vi "Control BrakeCoast[Conflict].vi"   [LabVIEW 2017]
uses:
  <vilib>/Rock Robotics/WPI/ThirdParty/Phoenix-LabVIEW/Motor Controller/Controls/CTRE_Phoenix_MotorControl_NeutralMode.ctl
types:
  T1 = cluster{"LinearAcceleration X":dbl, "LinearAcceleration Y":dbl, "LinearAcceleration Z":dbl}
  T2 = typedef "WPI_MotorControlDeviceRef.ctl" = cluster{"DeviceStatus":errorcluster, "Type":T3, "PWM":cluster{"PWM Channel":T4, "DeadBand":T5}, "CAN":cluster{"Device Number":u8, "SetOutput VI Ref":variant, "GetOutput VI Ref":variant, "Enable VI Ref":variant, "Disable VI Ref":variant, "Data":variant}, "Invert":bool, "DIO PWM":cluster{"PWM \"Enable\" Channel":T4, "DIOChannel":T6, "PWM Rate":dbl}}
  T3 = typedef "WPI_MotorControlType.ctl" = enum16{"PWM", "CAN", "DIO PWM"}
  T4 = typedef "FPGA_DIOPWMChannel.ctl" = enum8{"PWM 0", "PWM 1", "PWM 2", "PWM 3", "PWM 4", "PWM 5", "PWM 6", "PWM 7", "PWM 8", "PWM 9", "PWM MXP 0", "PWM MXP 1", "PWM MXP 2", "PWM MXP 3", "PWM MXP 4", "PWM MXP 5", "PWM MXP 6", "PWM MXP 7", "PWM MXP 8", "PWM MXP 9", "Invalid"}
  T5 = typedef "WPI_PWMDeadband.ctl" = cluster{"Name":string, "maxPositivePwm":i32, "minPositivePwm":i32, "centerPwm":i32, "maxNegativePwm":i32, "minNegativePwm":i32, "angularRange":u16}
  T6 = typedef "FPGA_DIOChannel.ctl" = enum8{"DIO 0", "DIO 1", "DIO 2", "DIO 3", "DIO 4", "DIO 5", "DIO 6", "DIO 7", "DIO 8", "DIO 9", "DIO MXP 0", "DIO MXP 1", "DIO MXP 2", "DIO MXP 3", "DIO MXP 4", "DIO MXP 5", "DIO MXP 6", "DIO MXP 7", "DIO MXP 8", "DIO MXP 9", "DIO MXP 10", "DIO MXP 11", "DIO MXP 12", "DIO MXP 13", "DIO MXP 14", "DIO MXP 15", "SPI Port CS1", "SPI Port CS2", "SPI Port CS3", "SPI Port MISO", "SPI Port MOSI", "Invalid"}
  T7 = typedef "CTRE_Phoenix_MotorControl_NeutralMode.ctl" = enum8{"EEPROMSetting", "Override to Coast", "Override to Brake"}
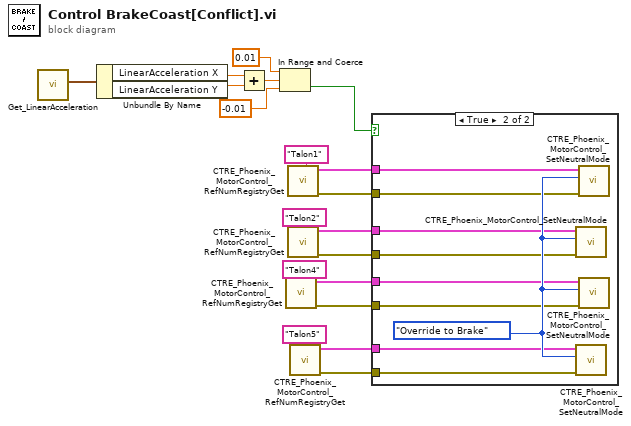
[diagram p0: block diagram]
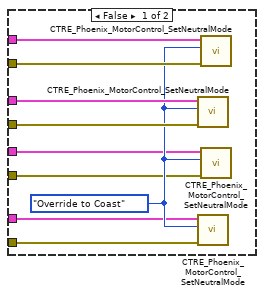
[diagram p2: hidden frame]
diagram:
  n1 = call <vilib>:"Get_LinearAcceleration.vi"() -> ("Linear Acceleration"=w17:T1)  [unwired: 11 in]
  n2 = Unbundle By Name(w17) -> ("LinearAcceleration X"=w18:dbl, "LinearAcceleration Y"=w19:dbl)
  n3 = Add(x=w18, y=w19) -> (x+y=w16:dbl)
  n4 = In Range and Coerce(upper limit=0.01, x=w16, lower limit=-0.01) -> (In Range?=w1:bool)  [unwired: 1 out]
  n5 = call <vilib>:"CTRE_Phoenix_MotorControl_RefNumRegistryGet.vi"("refnum name"="Talon4") -> ("error out"=w6:errorcluster, "PhoenixMotorControlDevRef"=w7:T2)  [unwired: 9 in]
  n6 = call <vilib>:"CTRE_Phoenix_MotorControl_RefNumRegistryGet.vi"("refnum name"="Talon1") -> ("error out"=w12:errorcluster, "PhoenixMotorControlDevRef"=w13:T2)  [unwired: 9 in]
  n7 = call <vilib>:"CTRE_Phoenix_MotorControl_RefNumRegistryGet.vi"("refnum name"="Talon2") -> ("error out"=w9:errorcluster, "PhoenixMotorControlDevRef"=w10:T2)  [unwired: 9 in]
  n8 = call <vilib>:"CTRE_Phoenix_MotorControl_RefNumRegistryGet.vi"("refnum name"="Talon5") -> ("error out"=w3:errorcluster, "PhoenixMotorControlDevRef"=w4:T2)  [unwired: 9 in]
  n9 = case shown="True" w1 {
    tunnel: w13 -> [w28 w36]
    tunnel: w12 -> [w27 w35]
    tunnel: w10 -> [w26 w34]
    tunnel: w9 -> [w25 w33]
    tunnel: w7 -> [w20 w32]
    tunnel: w6 -> [w21 w31]
    tunnel: w4 -> [w23 w30]
    tunnel: w3 -> [w22 w29]
    frame False {
      w24 = CTRE_Phoenix_MotorControl_NeutralMode."Override to Coast" ("Motor Control Neutral Mode")
      n10 = call <vilib>:"CTRE_Phoenix_MotorControl_SetNeutralMode.vi"("error in (no error)"=w25, "Motor Control Neutral Mode"=w24, "PhoenixMotorControlDevRef"=w26) -> ()  [unwired: 7 in, 2 out]
      n11 = call <vilib>:"CTRE_Phoenix_MotorControl_SetNeutralMode.vi"("error in (no error)"=w22, "Motor Control Neutral Mode"=w24, "PhoenixMotorControlDevRef"=w23) -> ()  [unwired: 7 in, 2 out]
      n12 = call <vilib>:"CTRE_Phoenix_MotorControl_SetNeutralMode.vi"("error in (no error)"=w27, "Motor Control Neutral Mode"=w24, "PhoenixMotorControlDevRef"=w28) -> ()  [unwired: 7 in, 2 out]
      n13 = call <vilib>:"CTRE_Phoenix_MotorControl_SetNeutralMode.vi"("error in (no error)"=w21, "Motor Control Neutral Mode"=w24, "PhoenixMotorControlDevRef"=w20) -> ()  [unwired: 7 in, 2 out]
    }
    frame True {
      w37 = CTRE_Phoenix_MotorControl_NeutralMode."Override to Brake" ("Motor Control Neutral Mode")
      n14 = call <vilib>:"CTRE_Phoenix_MotorControl_SetNeutralMode.vi"("error in (no error)"=w33, "Motor Control Neutral Mode"=w37, "PhoenixMotorControlDevRef"=w34) -> ()  [unwired: 7 in, 2 out]
      n15 = call <vilib>:"CTRE_Phoenix_MotorControl_SetNeutralMode.vi"("error in (no error)"=w29, "Motor Control Neutral Mode"=w37, "PhoenixMotorControlDevRef"=w30) -> ()  [unwired: 7 in, 2 out]
      n16 = call <vilib>:"CTRE_Phoenix_MotorControl_SetNeutralMode.vi"("error in (no error)"=w35, "Motor Control Neutral Mode"=w37, "PhoenixMotorControlDevRef"=w36) -> ()  [unwired: 7 in, 2 out]
      n17 = call <vilib>:"CTRE_Phoenix_MotorControl_SetNeutralMode.vi"("error in (no error)"=w31, "Motor Control Neutral Mode"=w37, "PhoenixMotorControlDevRef"=w32) -> ()  [unwired: 7 in, 2 out]
    }
  }
